vi "Actor Event.vi"(8 "Queue Mailbox":refnum<data-value>, 9 "Self Event Alias":string, 10 "Queue of Self Event":refnum<queue>, 11 "Event":refnum<class "Event.lvclass">) -> ()   [LabVIEW 2021, in "jettl.lvlib" / "Base Event.lvlib" / "Base Event.lvclass"]
uses:
  Base Event.lvclass
  Self Event/Self Event.lvlib
  Event/Event.lvclass
  jettl.lvlib
  jettl Msg Last Ack Created Event/jettl Msg Last Ack Created Event.lvlib
  C:/git/jettl/src/jettl/jettl/jettl.lvclass
  C:/git/jettl/src/jettl Msg Merge Error/jettl Msg Merge Error/jettl Msg Merge Error.lvclass
  C:/git/jettl/src/jettl/Event/Event.lvclass
  C:/git/jettl/src/jettl Msg Override Error/jettl Msg Override Error/jettl Msg Override Error.lvclass
  C:/git/jettl/src/jettl Msg Setup/jettl Msg Setup/jettl Msg Setup.lvclass
  C:/git/jettl/src/jettl Msg Teardown/jettl Msg Teardown/jettl Msg Teardown.lvclass
  C:/git/jettl/src/jettl/jettl Msg Last Ack Creator Queue/jettl Msg Last Ack Creator Queue/jettl Msg Last Ack Creator Queue.lvclass
  C:/git/jettl/src/jettl/Base Event/Base Event/Base Event.lvclass
  Msg Strategy/Msg Strategy.lvclass
  Queue Mailbox/Queue Mailbox/Queue Mailbox.lvclass
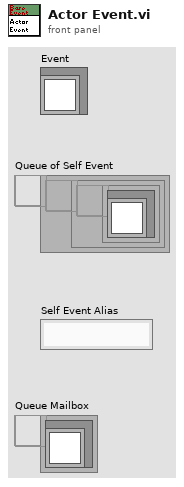
[diagram p1: front panel]
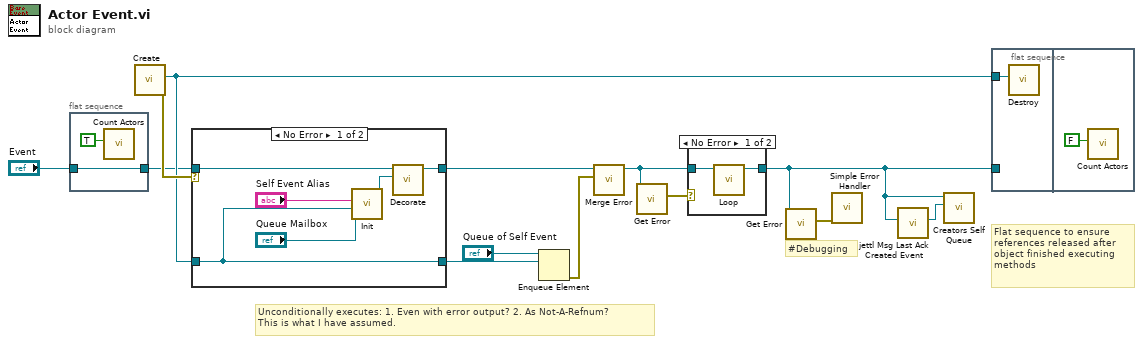
[diagram p0: block diagram]
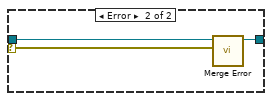
[diagram p2: hidden frame]
diagram:
  # "Flat sequence to ensure references released after object finished executing methods"
  # "#Debugging"
  # "Unconditionally executes: 1. Even with error output? 2. As Not-A-Refnum?\nThis is what I have assumed."
  n1 = flat-sequence {
    tunnel: [w14] -> w5
    tunnel: "Event" -> [w14]
    frame #0 {
      n2 = call "Count Actors.vi"("Increment?"=TRUE) -> ()  [unwired: 11 in]
    }
  }
  n3 = call "Create.vi"() -> ("error out"=w8:errorcluster, "Self Event"=w7:refnum<data-value>)  [unwired: 10 in]
  n4 = case shown="No Error" w8 {
    selector: w8 -> [_ w23]
    tunnel: [w19 w24] -> w11
    tunnel: w5 -> [w21 w22]
    tunnel: w7 -> [w16 _]
    tunnel: [w16 _] -> w10
    frame No Error {
      n5 = call "Init.vi"("Queue Mailbox"="Queue Mailbox", "Self Event"=w16, "Self Event Alias"="Self Event Alias") -> ("Base Event out"=w20:refnum<class "Base Event.lvclass">)  [unwired: 8 in]
      n6 = call-dynamic "Decorate.vi"("Event"=w20, "Event in"=w21) -> ("Event out"=w19:refnum<class "Event.lvclass">)  [unwired: 9 in]
    }
    frame Error {
      n7 = call-dynamic "Merge Error.vi"("Error"=w23, "jettl Msg Merge Error in"=w22) -> ("jettl Msg Merge Error out"=w24:refnum<class "Event.lvclass">)  [unwired: 9 in]
    }
  }
  n8 = Enqueue Element(queue="Queue of Self Event", element=w10) -> (error out=w12:errorcluster)  [unwired: 2 in, 2 out]
  n9 = call-dynamic "Merge Error.vi"("Error"=w12, "jettl Msg Merge Error in"=w11) -> ("jettl Msg Merge Error out"=w13:refnum<class "Event.lvclass">)  [unwired: 9 in]
  n10 = call-dynamic "Get Error.vi"("jettl in"=w13) -> ("Error"=w9:errorcluster)  [unwired: 10 in]
  n11 = case shown="No Error" w9 {
    tunnel: w13 -> [w26 w27]
    tunnel: [w25 w27] -> w1
    frame No Error {
      n12 = call-dynamic "Loop.vi"("Event in"=w26) -> ("Event out"=w25:refnum<class "Event.lvclass">)  [unwired: 10 in]
    }
    frame Error {
    }
  }
  n13 = call-dynamic "Get Error.vi"("jettl in"=w1) -> ("Error"=w3:errorcluster)  [unwired: 10 in]
  n14 = call <vilib>:"Simple Error Handler.vi"("error in (no error)"=w3) -> ()  [unwired: 4 in, 5 out]
  n15 = call "jettl Msg Last Ack Created Event.vi"("Event"=w1) -> ("Msg Strategy"=w2:refnum<class "Msg Strategy.lvclass">)  [unwired: 10 in]
  n16 = call-dynamic "Creators Self Queue.vi"("Msg Strategy"=w2, "Event in"=w1) -> ()  [unwired: 9 in, 1 out]
  n17 = flat-sequence {
    tunnel: w7 -> [w28]
    tunnel: w1 -> [_]
    frame #0 {
      n18 = call "Destroy.vi"("Self Event"=w28) -> ()  [unwired: 10 in, 1 out]
    }
    frame #1 {
      n19 = call "Count Actors.vi"("Increment?"=FALSE) -> ()  [unwired: 11 in]
    }
  }
